vi "Register Size Event.vi"(8 "error in (no error)":errorcluster, 11 "Terminal in":refnum<class "Terminal.lvclass">) -> (0 "error out":errorcluster, 2 "Size Event Reg":refnum<event-registration>, 3 "Terminal out":refnum<class "Terminal.lvclass">)   [LabVIEW 2020, in "Terminal.lvlib" / "Terminal.lvclass"]
uses:
  Terminal.lvclass
  Terminal.lvclass/Terminal.ctl
  <vilib>/Utility/miscctls.llb/LVBoundsTypeDef.ctl
  Size Event Data.ctl
  Terminal.lvlib
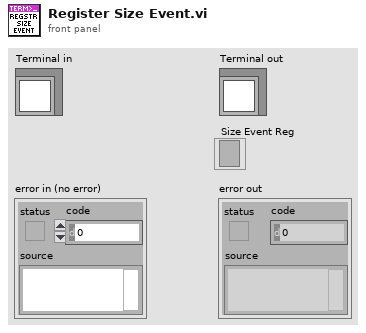
[diagram p1: front panel]
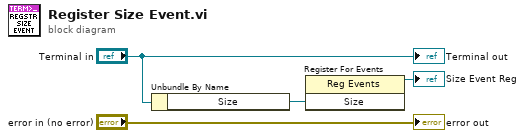
[diagram p0: block diagram]
diagram:
  n1 = Unbundle By Name("Terminal in") -> ("Size"=w2:refnum<user-event>)
  n2 = register-events(w2) -> (reference out=→"Size Event Reg":refnum<event-registration>)  [unwired: 2 in, 1 out]
  "error out" <- "error in (no error)"
  "Terminal out" <- "Terminal in"
